vi "Test Enumerate Camera Devices.vi"(8 "error in (no error)":errorcluster, 11 "Test Case In":refnum<class "50_Capture.lvclass">) -> (0 "error out":errorcluster, 3 "Test Case Out":refnum<class "50_Capture.lvclass">)   [LabVIEW 2020, in "test.lvlib" / "50_Capture.lvclass"]
uses:
  50_Capture.lvclass
  C:/Program Files (x86)/National Instruments/LabVIEW 2026/vi.lib/Astemes/LUnit/Test Case.lvclass
  <vilib>/Astemes/LUnit/Test Case.lvclass/Test Case.ctl
  <vilib>/Astemes/LUnit/Core/LUnit Test Case/Private/Append Fail Result.vi
  <vilib>/Astemes/LUnit/Core/LUnit Test Case/Private/Append Pass Result.vi
  <vilib>/Astemes/LUnit/Core/LUnit Test Case/Private/Run In UI.vi
  <vilib>/Utility/error.llb/Clear Errors.vi
  capture/capture.lvlib
  <vilib>/Astemes/LUnit/Test Case.lvclass
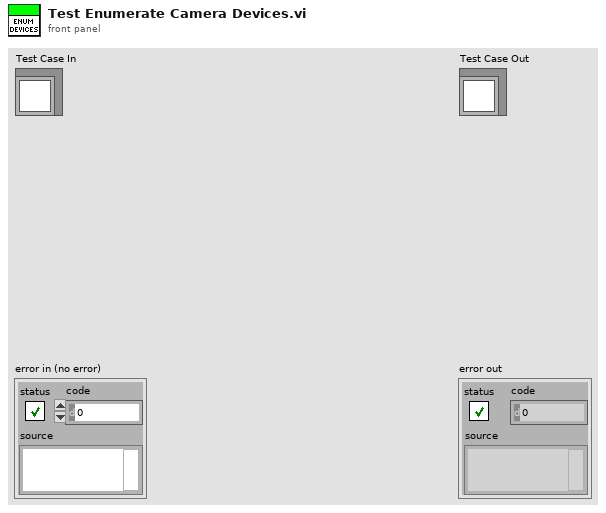
[diagram p1: front panel]
types:
  T1 = typedef "capture.lvlib/Stream.lvclass/Stream Specification.ctl" = cluster{"Size":T2, "FPS":T3}
  T2 = typedef "common.lvlib/Image Size (Integer).ctl" = cluster{"Width":u16, "Height":u16}
  T3 = typedef "capture.lvlib/Stream.lvclass/Frames per Second.ctl" = cluster{"Numerator":u32, "Denominator":u32}
  T4 = cluster{"ID":string, "Name":string, "Stream Specifications":T1[]}[]
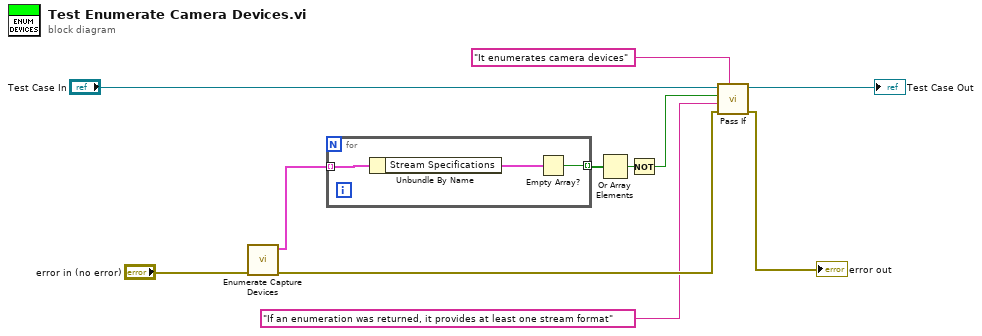
[diagram p0: block diagram]
diagram:
  n1 = call "Enumerate Capture Devices.vi"("error in (no error)"="error in (no error)") -> ("error out"=w7:errorcluster, "Devices"=w1:T4)  [unwired: 9 in]
  n2 = for {
    tunnel: w1 -> [w14] mode=indexing
    tunnel: [w12] -> w5 mode=indexing
    n3 = Unbundle By Name(w14) -> ("Stream Specifications"=w13:T1[])
    n4 = Empty Array?(array=w13) -> (empty?=w12:bool)
  }
  n5 = Or Array Elements(Boolean array=w5) -> (logical OR=w4:bool)
  n6 = Not(x=w4) -> (.not. x?=w2:bool)
  n7 = call <vilib>:"Pass If.vi"("Description"="It enumerates camera devices", "error in (no error)"=w7, "Message"="If an enumeration was returned, it provides at least one stream format", "Pass?"=w2, "LUnit Test Case In"="Test Case In") -> ("error out"=→"error out":errorcluster, "LUnit Test Case Out"=→"Test Case Out":refnum<class "50_Capture.lvclass">)  [unwired: 5 in]
